vi "Main.vi"(8 "error in":errorcluster, 11 "UGM BEEP in":refnum<class "UGM BEEP.lvclass">) -> (0 "error out":errorcluster, 3 "UGM BEEP out":refnum<class "UGM BEEP.lvclass">)   [LabVIEW 2024, in "UGM BEEP.lvclass"]
doc: "The <b>Queued Message Handler</b> of the Worker that owns this VI."
uses:
  UGM BEEP.lvclass
  UGM BEEP.lvclass/UGM BEEP.ctl
  <vilib>/Python/Open Venv Python Session.vi
  rqp_UGM BEEP.ctl
panel:
  in  "Data in":T1={"Frequency"=1500, "Duration"=300}
  in  "Button":bool
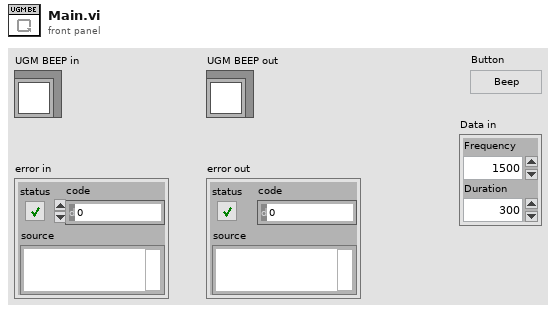
[diagram p1: front panel]
types:
  T1 = typedef "UGM BEEP.lvclass/rqp_UGM BEEP.ctl" = cluster{"Frequency":u32, "Duration":u32}
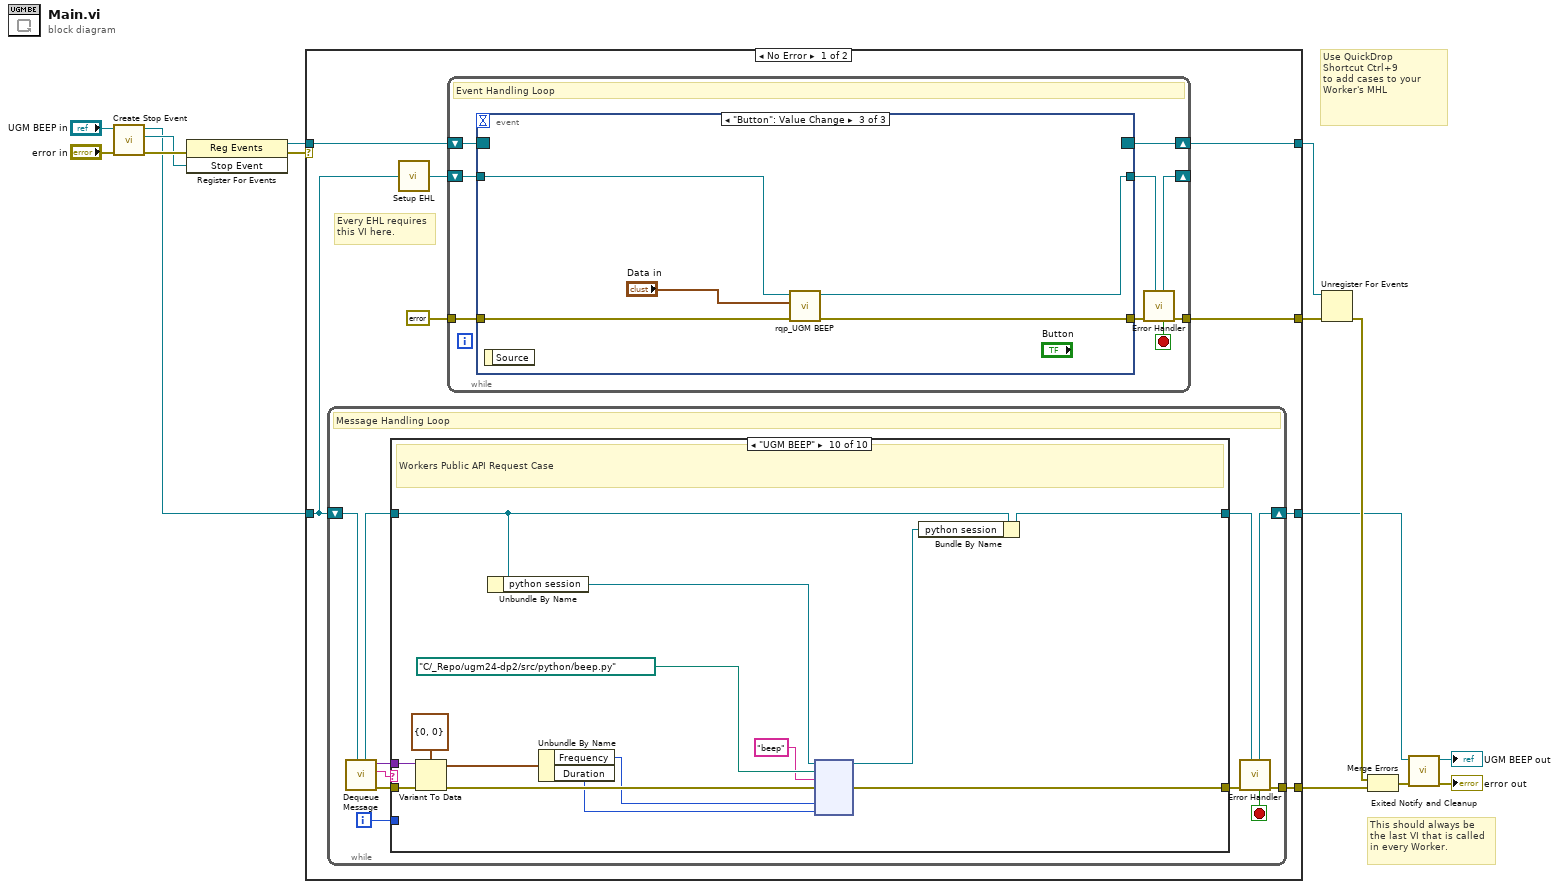
[diagram p0: block diagram]
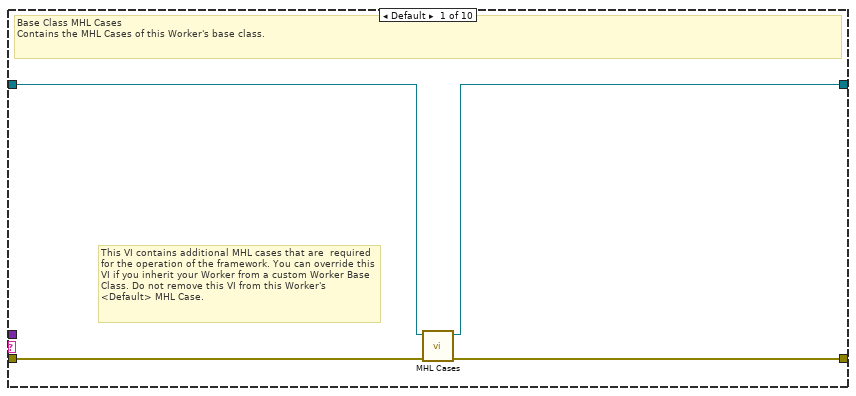
[diagram p2: hidden frame]
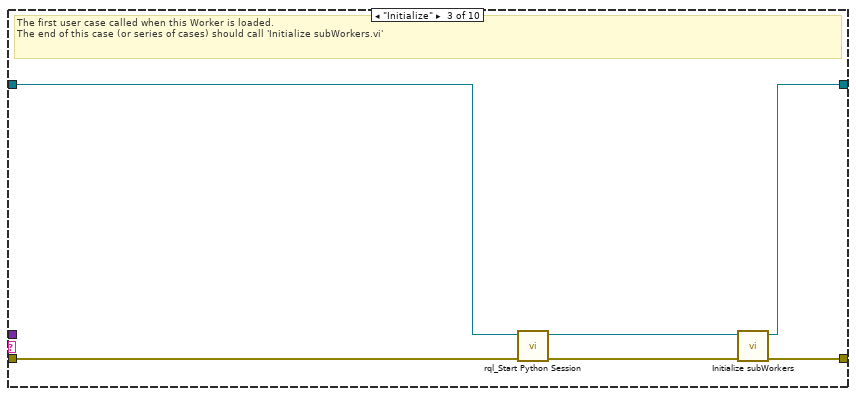
[diagram p4: hidden frame]
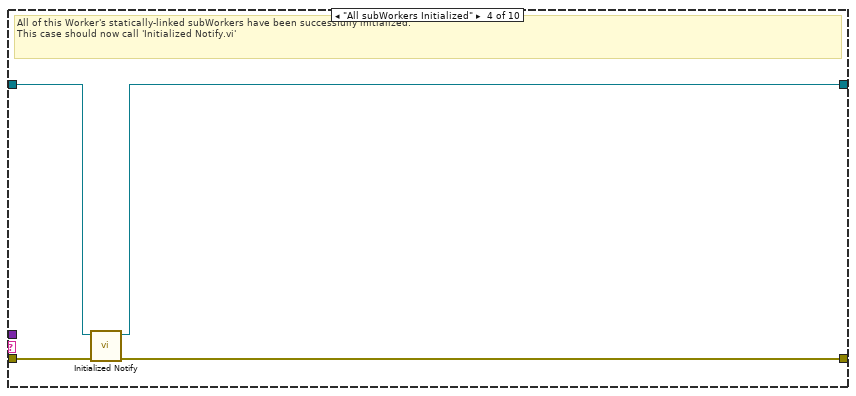
[diagram p5: hidden frame]
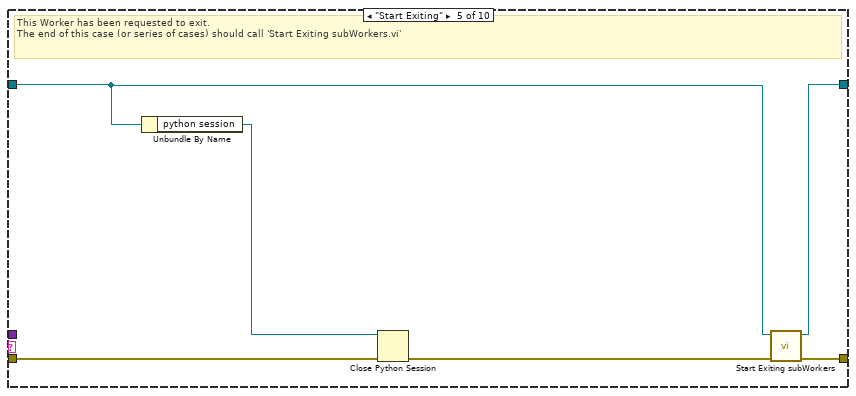
[diagram p6: hidden frame]
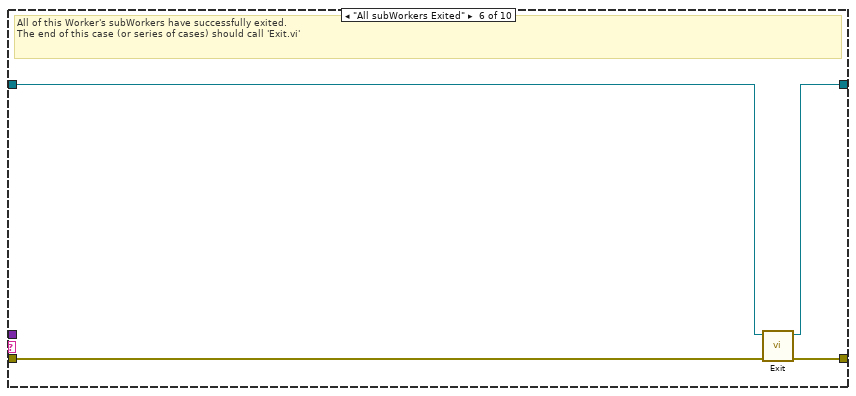
[diagram p7: hidden frame]
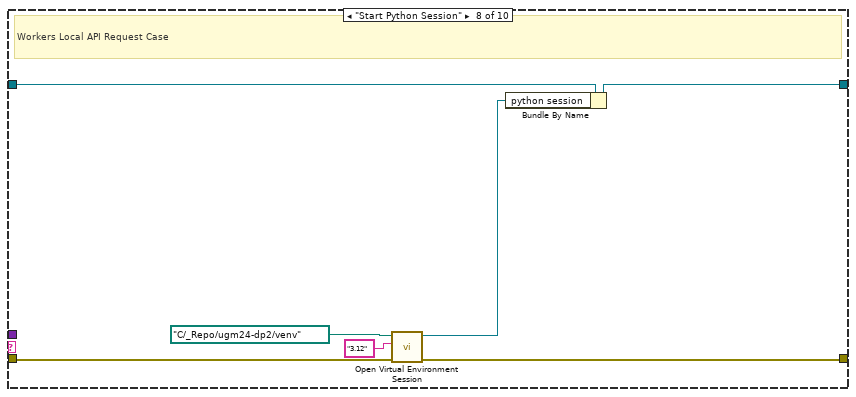
[diagram p9: hidden frame]
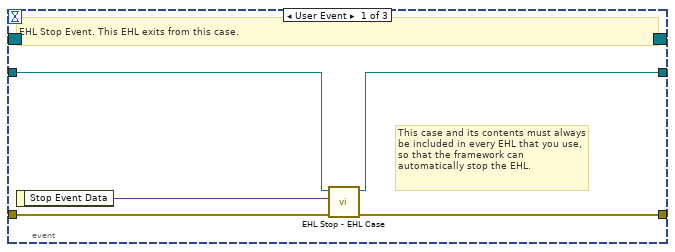
[diagram p11: hidden frame]
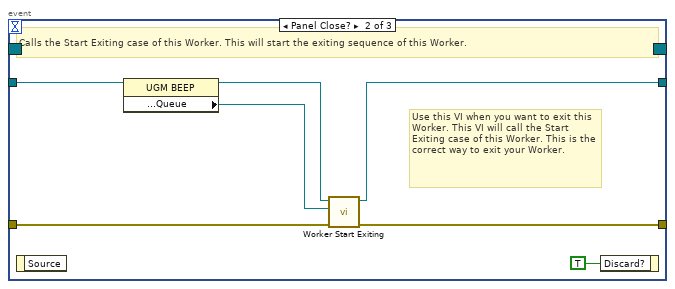
[diagram p12: hidden frame]
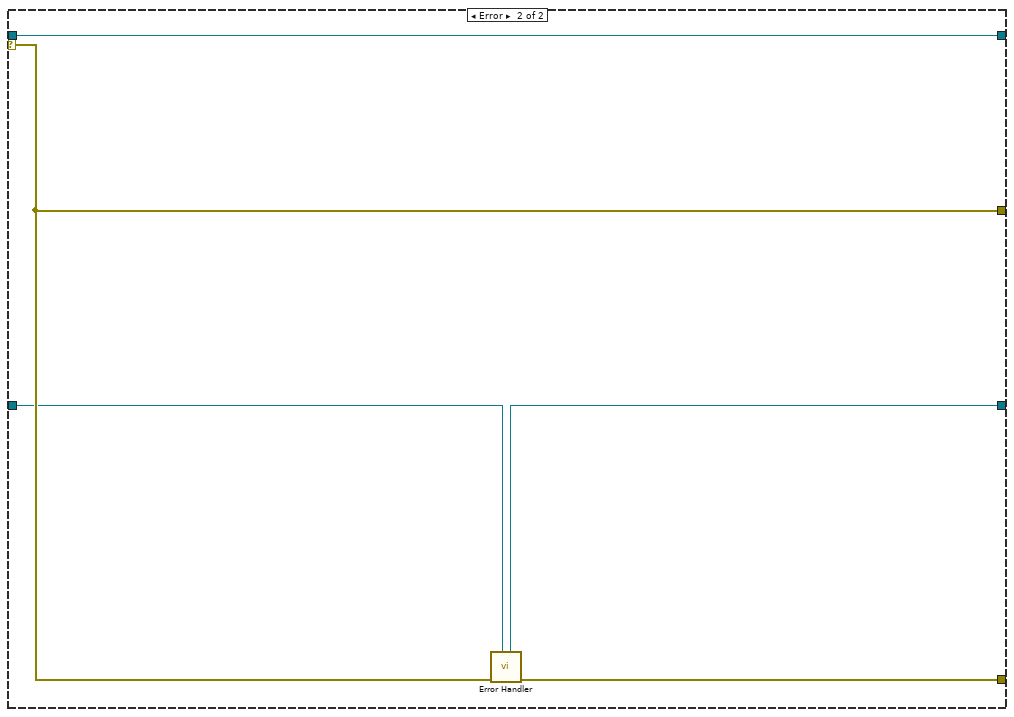
[diagram p13: hidden frame]
diagram:
  # "Use QuickDrop\nShortcut Ctrl+9\nto add cases to your\nWorker's MHL"
  # "This should always be the last VI that is called in every Worker."
  n1 = call-dynamic "Create Stop Event.vi"("error in"="error in", "Worker"="UGM BEEP in") -> ("error out"=w10:errorcluster, "Stop Event"=w7:refnum<user-event>, "Worker out"=w4:refnum<class "UGM BEEP.lvclass">)  [unwired: 7 in]
  n2 = register-events(error in=w10, w7) -> (reference out=w9:refnum<event-registration>, error out=w1:errorcluster)  [unwired: 1 in]
  n3 = case shown="No Error" w1 {
    tunnel: w4 -> [w18 w113]
    tunnel: [w16 w114] -> w8
    tunnel: w9 -> [w23 w115]
    tunnel: [w20 w116] -> w14
    tunnel: [w22 w115] -> w13
    tunnel: [w17 w112] -> w11
    selector: w1 -> [_ w116]
    frame No Error {
      # "Every EHL requires\nthis VI here."
      n4 = while {
        shift-right: [w32] -> w17
        shift-left: w18 -> [w34]
        tunnel: [w33] -> w16
        i -> [w25]
        stop <- w26 stop-if-true
        # "Message Handling Loop"
        n5 = call-dynamic "Dequeue Message.vi"("Worker"=w34) -> ("error out"=w31:errorcluster, "Case out"=w27:string, "Data out"=w24:variant, "Worker out"=w29:refnum<class "UGM BEEP.lvclass">)  [unwired: 6 in, 1 out]
        n6 = case "Worker MHL Case Structure (DO NOT CHANGE LABEL NAME)" shown="\"UGM BEEP\"" w27 {
          tunnel: w31 -> [w38 w39 w41 w48 w54 w60 w62 w66 w71 w85]
          tunnel: [w37 w39 w46 w47 w56 w59 w62 w65 w71 w79] -> w30
          tunnel: w29 -> [w36 w40 w42 w50 w53 w58 w61 w69 w70 w80]
          tunnel: [w35 w40 w45 w49 w55 w57 w61 w64 w70 w76] -> w28
          tunnel: w25 -> [_ _ _ _ _ _ _ _ _ _]
          tunnel: w24 -> [_ _ _ _ _ _ _ _ _ w82]
          frame Default {
            # "This VI contains additional MHL cases that are  required for the operation of the framework. You can override this VI if you inherit your Worker from a custom Worker Base Class. Do not remove this VI from this Worker's <Default> MHL Case."
            # "Base Class MHL Cases\nContains the MHL Cases of this Worker's base class."
            n7 = call-dynamic "MHL Cases.vi"("error in"=w38, "Worker in"=w36) -> ("error out"=w37:errorcluster, "Worker out"=w35:refnum<class "UGM BEEP.lvclass">)  [unwired: 8 in]
          }
          frame "------------ FRAMEWORK CASES -----------" {
            # "Start of Workers Framework Cases"
          }
          frame "Initialize" {
            # "The first user case called when this Worker is loaded.\nThe end of this case (or series of cases) should call 'Initialize subWorkers.vi'"
            n8 = call "rql_Start Python Session.vi"("error in"=w41, "CPU Percent in"=w42) -> ("error out"=w44:errorcluster, "dup CPU Percent out"=w43:refnum<class "UGM BEEP.lvclass">)  [unwired: 8 in]
            n9 = call-dynamic "Initialize subWorkers.vi"("error in"=w44, "Worker"=w43) -> ("error out"=w46:errorcluster, "dup Worker out"=w45:refnum<class "UGM BEEP.lvclass">)  [unwired: 8 in]
          }
          frame "All subWorkers Initialized" {
            # "All of this Worker's statically-linked subWorkers have been successfully initialized.\nThis case should now call 'Initialized Notify.vi'"
            n10 = call-dynamic "Initialized Notify.vi"("error in"=w48, "Worker"=w50) -> ("error out"=w47:errorcluster, "dup Worker out"=w49:refnum<class "UGM BEEP.lvclass">)  [unwired: 8 in]
          }
          frame "Start Exiting" {
            # "This Worker has been requested to exit. \nThe end of this case (or series of cases) should call 'Start Exiting subWorkers.vi'"
            n11 = Unbundle By Name(w53) -> ("python session"=w51:refnum<k35>)
            n12 = Close Python Session(session in=w51, error in=w54) -> (11:w52:errorcluster)
            n13 = call-dynamic "Start Exiting subWorkers.vi"("error_in"=w52, "Worker"=w53) -> ("error out"=w56:errorcluster, "dup Worker out"=w55:refnum<class "UGM BEEP.lvclass">)  [unwired: 8 in]
          }
          frame "All subWorkers Exited" {
            # "All of this Worker's subWorkers have successfully exited. \nThe end of this case (or series of cases) should call 'Exit.vi'"
            n14 = call-dynamic "Exit.vi"("error_in"=w60, "Worker"=w58) -> ("error out"=w59:errorcluster, "dup Worker out"=w57:refnum<class "UGM BEEP.lvclass">)  [unwired: 8 in]
          }
          frame "------------- LOCAL API CASES -------------" {
            # "Start of Workers Local API Cases"
          }
          frame "Start Python Session" {
            # "Workers Local API Request Case"
            n15 = call-poly <vilib>:"Open Virtual Environment Session.vi"("error in (no error)"=w66, "Python version"="3.12", "Env path"=path "C:/_Repo/ugm24-dp2/venv") -> ("error out"=w65:errorcluster, "session out"=w63:refnum<k35>)  [unwired: 7 in]
            n16 = Bundle By Name(cluster=w69, "python session"=w63) -> (w64:refnum<class "UGM BEEP.lvclass">)
          }
          frame "------------- PUBLIC API CASES -------------" {
            # "Start of Workers Public API Cases"
          }
          frame "UGM BEEP" {
            # "Workers Public API Request Case"
            n17 = Variant To Data(error in=w85, type=T1 {"Frequency"=0, "Duration"=0} ("Data"), Variant=w82) -> (data=w81:T1, error out=w84:errorcluster)
            n18 = Unbundle By Name(w80) -> ("python session"=w78:refnum<k35>)
            n19 = Unbundle By Name(w81) -> ("Frequency"=w73:u32, "Duration"=w72:u32)
            n20 = node(w78, path "C:/_Repo/ugm24-dp2/src/python/beep.py" ("module path"), "beep", w84, w73, w72) -> (w75:refnum<k35>, w79:errorcluster)  [unwired: 4 in, 2 out]
            n21 = Bundle By Name(cluster=w80, "python session"=w75) -> (w76:refnum<class "UGM BEEP.lvclass">)
          }
        }
        n22 = call-dynamic "Error Handler.vi"("Worker"=w28, "error_in"=w30) -> ("error out"=w33:errorcluster, "Stop Loop"=w26:bool, "Worker out"=w32:refnum<class "UGM BEEP.lvclass">)  [unwired: 7 in]
      }
      n23 = call-dynamic "Setup EHL.vi"("Worker"=w18) -> ("Worker out"=w19:refnum<class "UGM BEEP.lvclass">)  [unwired: 14 in]
      n24 = while "Event Handling Loop" {
        shift-right: [w94] -> w22
        shift-left: w23 -> [w93]
        tunnel: [w89] -> w20
        tunnel: errorcluster {"status"=FALSE, "code"=0, "source"=""} ("error constant") -> [w91]
        shift-right: [w87] -> _
        shift-left: w19 -> [w92]
        stop <- w86 stop-if-true
        # "Event Handling Loop"
        n25 = event shown="[2] \"Button\": Value Change" {
          selector: w93 -> [_ _ _]
          dyn-events: [_ _ _] -> w94
          timeout: _ -> [_ _ _]
          tunnel: [w98 w105 w110] -> w90
          tunnel: w91 -> [w99 w104 w111]
          tunnel: w92 -> [w97 w103 w109]
          tunnel: [w96 w102 w108] -> w88
          event User Event {
            # "This case and its contents must always be included in every EHL that you use, so that the framework can automatically stop the EHL."
            # "EHL Stop Event. This EHL exits from this case."
            n26 = event-data() -> ("Stop Event Data"=w95:variant)  [unwired: 1 in]
            n27 = call-dynamic "EHL Stop - EHL Case.vi"("error in"=w99, "Stop Event Data"=w95, "Worker"=w97) -> ("error out"=w98:errorcluster, "Worker out"=w96:refnum<class "UGM BEEP.lvclass">)  [unwired: 7 in]
          }
          event Panel Close? {
            # "Use this VI when you want to exit this Worker. This VI will call the Start Exiting case of this Worker. This is the correct way to exit your Worker."
            # "Calls the Start Exiting case of this Worker. This will start the exiting sequence of this Worker."
            n28 = event-data() -> ()  [unwired: 1 in, 1 out]
            n29 = property class="UGM BEEP"(reference=w103) -> (reference out=w101:refnum<class "UGM BEEP.lvclass">, "Accessors:Read:Public API:Queue"=w100:refnum<class "Message Queue.lvclass">)  [unwired: 1 in, 1 out]
            n30 = call-dynamic "Worker Start Exiting.vi"("error_in"=w104, "Message Queue"=w100, "Worker"=w101) -> ("error out"=w105:errorcluster, "dup Worker out"=w102:refnum<class "UGM BEEP.lvclass">)  [unwired: 7 in]
            n31 = event-data("Discard?"=TRUE) -> ()  [unwired: 1 in, 1 out]
          }
          event "Button": Value Change {
            n32 = event-data() -> ()  [unwired: 1 in, 1 out]
            n33 = call "rqp_UGM BEEP.vi"("error in"=w111, "Data in"="Data in", "UGM BEEP in"=w109) -> ("error out"=w110:errorcluster, "dup UGM BEEP out"=w108:refnum<class "UGM BEEP.lvclass">)  [unwired: 6 in, 1 out]
          }
        }
        n34 = call-dynamic "Error Handler.vi"("Worker"=w88, "error_in"=w90) -> ("error out"=w89:errorcluster, "Stop Loop"=w86:bool, "Worker out"=w87:refnum<class "UGM BEEP.lvclass">)  [unwired: 7 in]
      }
    }
    frame Error {
      n35 = call-dynamic "Error Handler.vi"("Worker"=w113, "error_in"=w116) -> ("error out"=w114:errorcluster, "Worker out"=w112:refnum<class "UGM BEEP.lvclass">)  [unwired: 7 in, 1 out]
    }
  }
  n36 = Unregister For Events(event registration refnum=w13, error in=w14) -> (error out=w15:errorcluster)
  n37 = Merge Errors(w15, w8) -> (w12:errorcluster)
  n38 = call-dynamic "Exited Notify and Cleanup.vi"("error_in"=w12, "Worker"=w11) -> ("error out"=→"error out":errorcluster, "dup Worker out"=→"UGM BEEP out":refnum<class "UGM BEEP.lvclass">)  [unwired: 8 in]
